vi "Configure Power Measurement List TX Increment Timing.vi"(8 "error in (no error)":errorcluster, 9 "Timing (Step)":i32(ring) items=["Step", "Center"], 10 "Instance (1)":i32=1, 11 "VISA resource name":refnum<visa-resource-name>) -> (0 "error out":errorcluster, 3 "VISA resource name out":refnum<visa-resource-name>)   [LabVIEW 2020, in "Rohde&Schwarz CMXP GPRF.lvlib"]
doc: "Specifies the timing of the generated power trigger.\n\nAttribute:\nRSCMXPGPRF_ATTR_POWER_MEASUREMENT_LIST_TX_INCREMENT_TIMING\n\nRemote-control command:\nCONFigure:GPRF:MEAS<i>:POWer:LIST:TXITiming"
uses:
  <instrlib>/Rohde&Schwarz CMXP GPRF/Rohde&Schwarz CMXP GPRF.lvlib
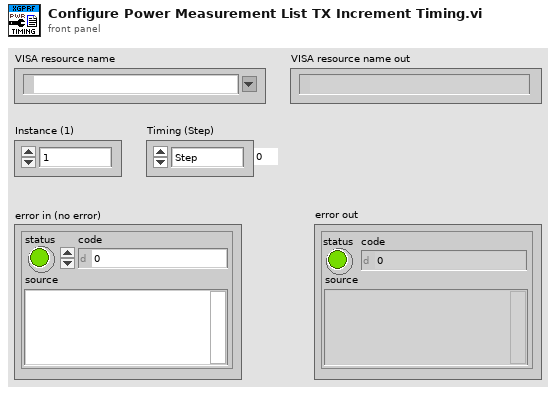
[diagram p1: front panel]
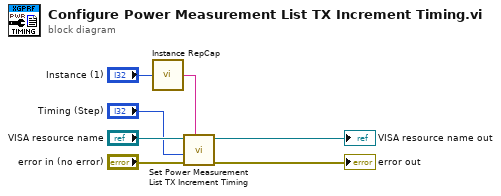
[diagram p0: block diagram]
diagram:
  n1 = call <instrlib>:"Instance RepCap.vi"("Instance in"="Instance (1)") -> ("Instance out"=w7:string)
  n2 = call "Set Power Measurement List TX Increment Timing"("Repeated Capabilities"=w7, "error in (no error)"="error in (no error)", "Power Measurement List TX Increment Timing (0 - Step)"="Timing (Step)", "instrument handle"="VISA resource name") -> ("error out"=→"error out":errorcluster, "instrument handle out"=→"VISA resource name out":refnum<visa-resource-name>)  [unwired: 6 in]
